vi "Marshal.vi"(8 "error in (no error)":errorcluster, 11 "Tag in":refnum<class "Proto Type Data Base.lvclass">) -> (0 "error out":errorcluster, 2 "Buffer":u8[](array[numeric]), 3 "Tag out":refnum<class "Proto Type Data Base.lvclass">)   [LabVIEW 2020, in "Protobuf RAW.lvlib" / "Proto Type Data Base.lvclass"]
uses:
  Proto Type Data Base.lvclass
  Proto Type Data Base.lvclass/Proto Type Data Base.ctl
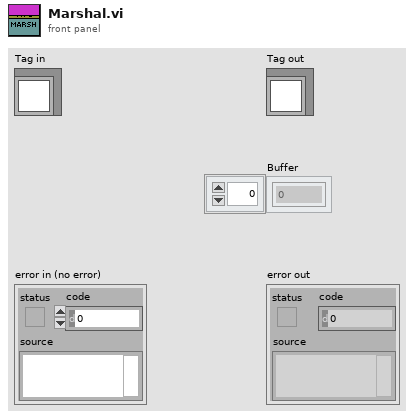
[diagram p1: front panel]
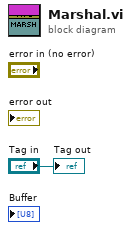
[diagram p0: block diagram]
diagram:
  "Tag out" <- "Tag in"
